vi "Get Last Data.vi"(0 "Lifter_motor in":refnum<class "Lifter_motor.lvclass">, 11 "error in (no error)":errorcluster) -> (4 "Lifter_motor out":refnum<class "Lifter_motor.lvclass">, 6 "Updated with new data":bool, 8 "Step distance":dbl, 10 "ADC Distance":dbl, 15 "error out":errorcluster)   [LabVIEW 2019, in "Lifter_motor.lvclass"]
uses:
  Lifter_motor.lvclass
  Lifter_motor.lvclass/Lifter_motor.ctl
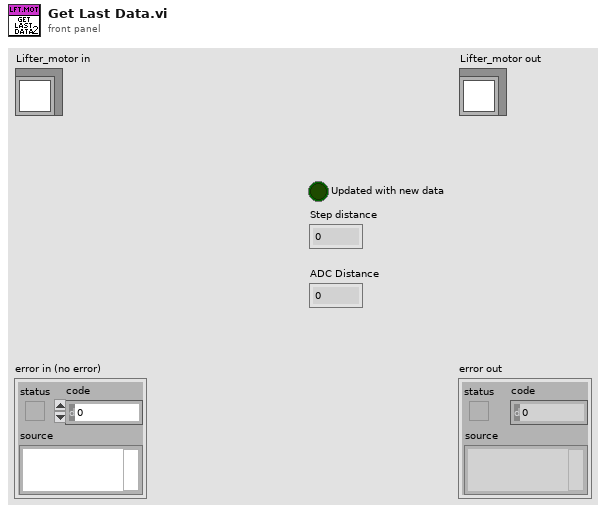
[diagram p1: front panel]
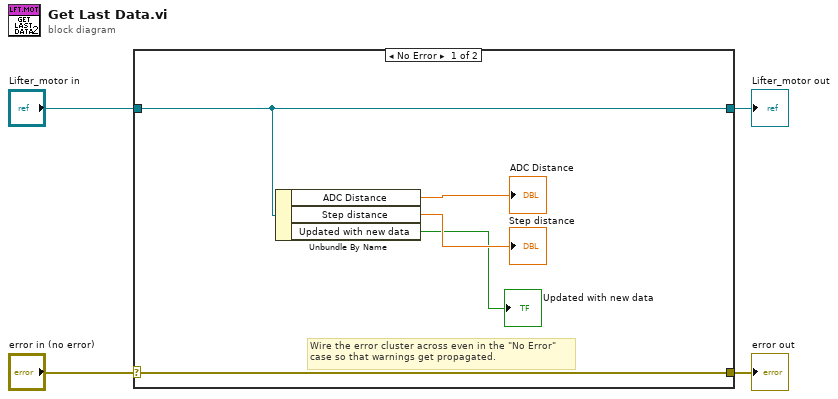
[diagram p0: block diagram]
diagram:
  n1 = case shown="No Error" "error in (no error)" {
    selector: "error in (no error)" -> [w9 w11]
    tunnel: [w9 w11] -> w3
    tunnel: [w8 w10] -> w1
    tunnel: "Lifter_motor in" -> [w8 w10]
    frame No Error {
      # "Wire the error cluster across even in the \"No Error\"\ncase so that warnings get propagated."
      n2 = Unbundle By Name(w8) -> ("ADC Distance"=→"ADC Distance":dbl, "Step distance"=→"Step distance":dbl, "Updated with new data"=→"Updated with new data":bool)
    }
    frame Error {
    }
  }
  "error out" <- w3
  "Lifter_motor out" <- w1
